vi "IR Emitter Test.vi"(5 "Test Configuration":T1, 8 "error in (no error)":errorcluster, 11 "Session Handle in":T8) -> (0 "error out":errorcluster, 1 "Failure Reason":string, 2 "Passed?":bool, 3 "Session Handle out":T8)   [LabVIEW 2015, in "PAS.lvclass"]
uses:
  PAS.lvclass
  Typedefs/Session Handle.ctl
  Tests/Controls/Test Configuration.ctl
  Tests/Controls/Vacuum Test.ctl
  Tests/Controls/Test Timing.ctl
  Tests/Controls/Vaccum Thresholds.ctl
  Tests/Controls/Helium Test.ctl
  Tests/Controls/Helium Thresholds.ctl
  Tests/Controls/Functional Test.ctl
  Typedefs/Emitter Power.ctl
  Typedefs/Valves.ctl
panel:
  out "Passed?":bool
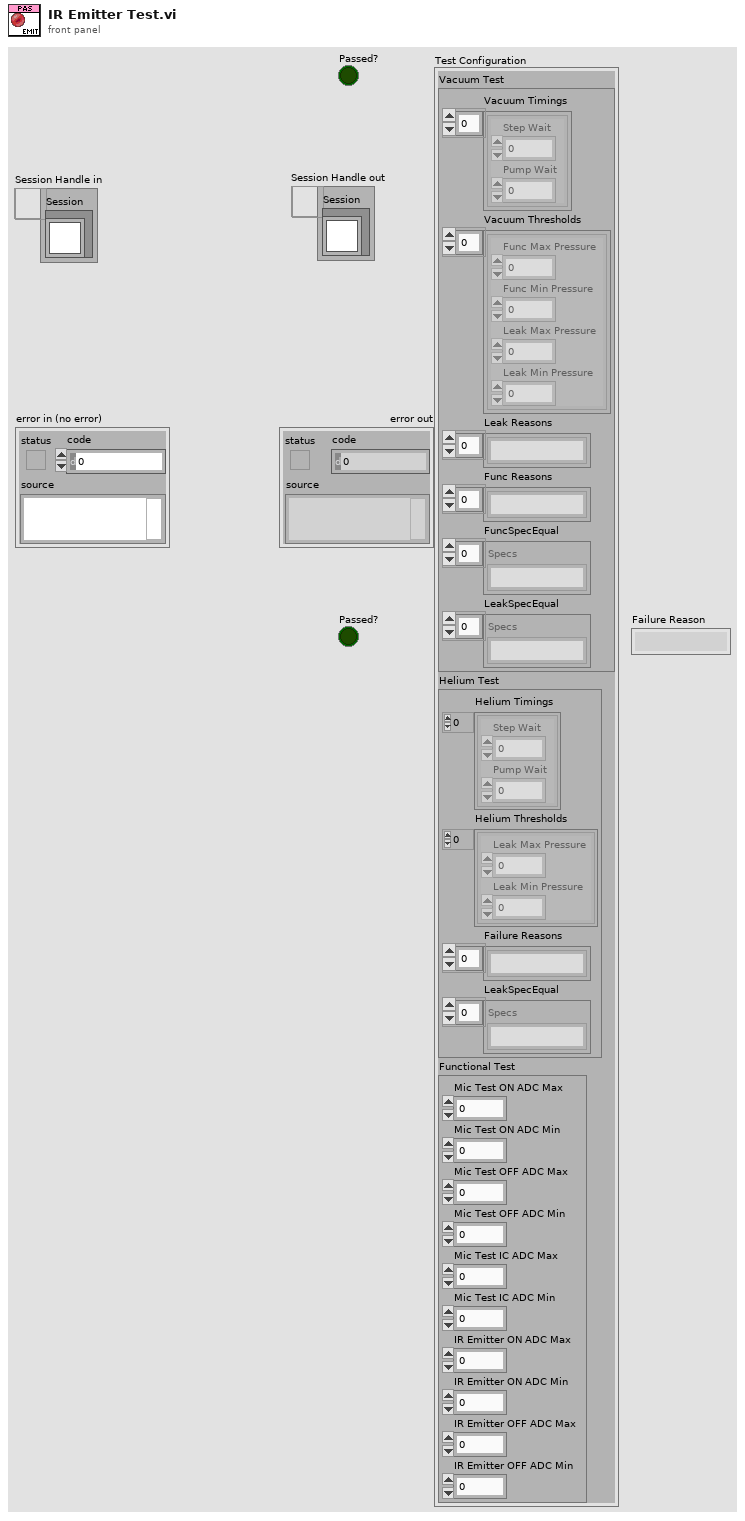
[diagram p1: front panel]
types:
  T1 = typedef "Test Configuration.ctl" = cluster{"Vacuum Test":T2, "Helium Test":T5, "Functional Test":T7}
  T2 = typedef "Vacuum Test.ctl" = cluster{"Vacuum Timings":T3[], "Vacuum Thresholds":T4[], "Leak Reasons":string[], "Func Reasons":string[], "FuncSpecEqual":string[], "LeakSpecEqual":string[]}
  T3 = typedef "Test Timing.ctl" = cluster{"Step Wait":dbl, "Pump Wait":dbl}
  T4 = typedef "Vaccum Thresholds.ctl" = cluster{"Func Max Pressure":dbl, "Func Min Pressure":dbl, "Leak Max Pressure":dbl, "Leak Min Pressure":dbl}
  T5 = typedef "Helium Test.ctl" = cluster{"Helium Timings":T3[], "Helium Thresholds":T6[], "Failure Reasons":string[], "LeakSpecEqual":string[]}
  T6 = typedef "Helium Thresholds.ctl" = cluster{"Leak Max Pressure":dbl, "Leak Min Pressure":dbl}
  T7 = typedef "Functional Test.ctl" = cluster{"Mic Test ON ADC Max":dbl, "Mic Test ON ADC Min":dbl, "Mic Test OFF ADC Max":dbl, "Mic Test OFF ADC Min":dbl, "Mic Test IC ADC Max":dbl, "Mic Test IC ADC Min":dbl, "IR Emitter ON ADC Max":dbl, "IR Emitter ON ADC Min":dbl, "IR Emitter OFF ADC Max":dbl, "IR Emitter OFF ADC Min":dbl}
  T8 = typedef "PAS.lvclass/Session Handle.ctl" = refnum<data-value>
  T9 = typedef "PAS.lvclass/Valves.ctl" = u16
  T10 = typedef "PAS.lvclass/Emitter Power.ctl" = u16
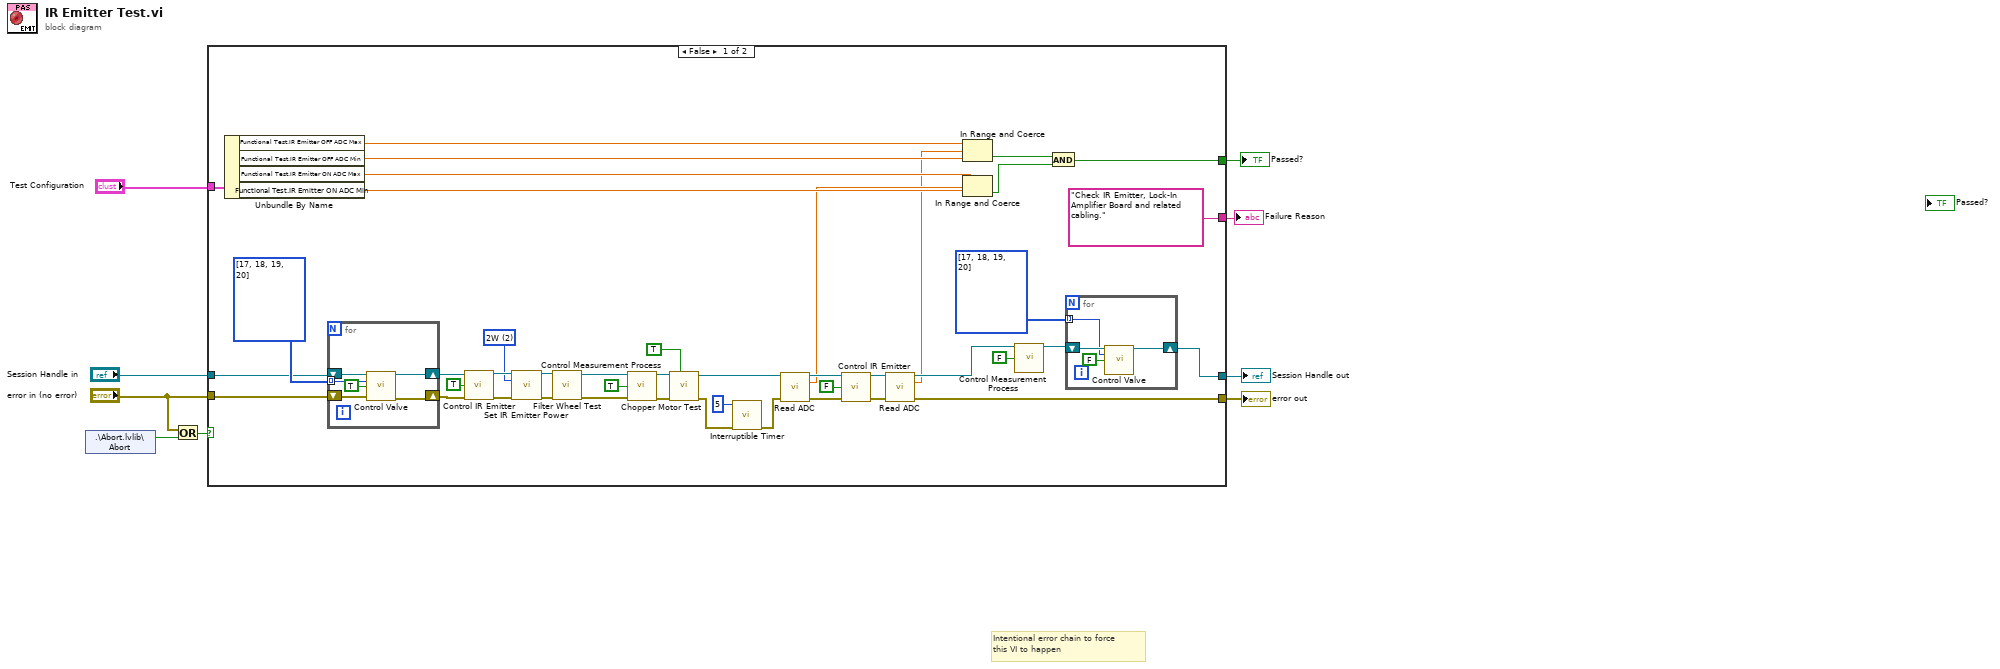
[diagram p0: block diagram]
diagram:
  # "Intentional error chain to force\nthis VI to happen"
  n1 = shared-variable ".\\Abort.lvlib\\Abort"() -> (w3:bool)  [unwired: 1 in, 1 out]
  n2 = Or(x="error in (no error)", y=w3) -> (x .or. y?=w4:bool)
  n3 = case shown="False" w4 {
    tunnel: "error in (no error)" -> [w52 w63]
    tunnel: [w42 w64] -> w9
    tunnel: "Session Handle in" -> [w41 w64]
    tunnel: "Test Configuration" -> [w40 _]
    tunnel: [w20 w63] -> w6
    tunnel: [w11 _] -> w5
    tunnel: ["Check IR Emitter, Lock-In Amplifier Board and related cabling." ("t") _] -> w1
    frame False {
      w22 = T9[] [17, 18, 19, 20] items=["PV1"=17, "PV2"=18, "PV3"=19, "PV4"=20]
      w45 = T10 2 items=["2W"=2, "3W"=3, "4W"=4, "5W"=5] ("Emitter Power")
      w51 = T9[] [17, 18, 19, 20] items=["PV1"=17, "PV2"=18, "PV3"=19, "PV4"=20]
      n4 = Unbundle By Name(w40) -> ("Functional Test.IR Emitter OFF ADC Max"=w16:dbl, "Functional Test.IR Emitter OFF ADC Min"=w15:dbl, "Functional Test.IR Emitter ON ADC Max"=w19:dbl, "Functional Test.IR Emitter ON ADC Min"=w18:dbl)
      n5 = for {
        shift-right: [w58] -> w50
        shift-left: w41 -> [w62]
        shift-right: [w59] -> w49
        shift-left: w52 -> [w60]
        tunnel: w51 -> [w61] mode=indexing
        n6 = call "Control Valve.vi"("Session Handle in"=w62, "Valves"=w61, "Energize?"=TRUE, "error in (no error)"=w60) -> ("Session Handle out"=w58:T8, "error out"=w59:errorcluster)  [unwired: 8 in, 2 out]
      }
      n7 = call "Control IR Emitter.vi"("Session Handle in"=w50, "Start?"=TRUE, "error in (no error)"=w49) -> ("Session Handle out"=w47:T8, "error out"=w46:errorcluster)  [unwired: 9 in, 2 out]
      n8 = call "Set IR Emitter Power.vi"("Session Handle in"=w47, "Emitter Power"=w45, "error in (no error)"=w46) -> ("Session Handle out"=w39:T8, "error out"=w38:errorcluster)  [unwired: 10 in, 1 out]
      n9 = call "Filter Wheel Test.vi"("error in (no error)"=w38, "Session Handle in"=w39) -> ("error out"=w29:errorcluster, "Session Handle out"=w30:T8)  [unwired: 7 in, 1 out]
      n10 = call "Control Measurement Process.vi"("Session Handle in"=w30, "Start?"=TRUE, "error in (no error)"=w29) -> ("Session Handle out"=w36:T8, "error out"=w35:errorcluster)  [unwired: 9 in, 2 out]
      n11 = call "Chopper Motor Test.vi"("Measurement Started?"=TRUE, "error in (no error)"=w35, "Session Handle in"=w36) -> ("error out"=w34:errorcluster, "Session Handle out"=w31:T8)  [unwired: 6 in, 1 out]
      n12 = call "Interruptible Timer.vi"("error in (no error)"=w34, "Wait (s)"=5) -> ("error out"=w32:errorcluster)  [unwired: 7 in, 2 out]
      n13 = call "Read ADC.vi"("Session Handle in"=w31, "error in (no error)"=w32) -> ("Session Handle out"=w27:T8, "ADC"=w17:dbl, "error out"=w26:errorcluster)  [unwired: 10 in, 1 out]
      n14 = call "Control IR Emitter.vi"("Session Handle in"=w27, "Start?"=FALSE, "error in (no error)"=w26) -> ("Session Handle out"=w24:T8, "error out"=w23:errorcluster)  [unwired: 9 in, 2 out]
      n15 = call "Read ADC.vi"("Session Handle in"=w24, "error in (no error)"=w23) -> ("Session Handle out"=w21:T8, "ADC"=w14:dbl, "error out"=w20:errorcluster)  [unwired: 10 in, 1 out]
      n16 = In Range and Coerce(upper limit=w16, x=w14, lower limit=w15) -> (In Range?=w13:bool)  [unwired: 1 out]
      n17 = In Range and Coerce(upper limit=w19, x=w17, lower limit=w18) -> (In Range?=w12:bool)  [unwired: 1 out]
      n18 = call "Control Measurement Process.vi"("Session Handle in"=w21, "Start?"=FALSE) -> ("Session Handle out"=w43:T8)  [unwired: 10 in, 3 out]
      n19 = And(x=w13, y=w12) -> (x .and. y?=w11:bool)
      n20 = for {
        shift-right: [w55] -> w42
        shift-left: w43 -> [w56]
        tunnel: w22 -> [w53] mode=indexing
        n21 = call "Control Valve.vi"("Session Handle in"=w56, "Valves"=w53, "Energize?"=FALSE) -> ("Session Handle out"=w55:T8)  [unwired: 9 in, 3 out]
      }
    }
    frame True {
    }
  }
  "error out" <- w6
  "Session Handle out" <- w9
  "Passed?" <- w5
  "Failure Reason" <- w1
